vi "Serial_sendot_v7 2.vi"(8 "Numeric 2":i32=20, 9 "VISA resource name":refnum<visa-resource-name>, 10 "Arduino":bool) -> (1 "Array":dbl[](array[numeric]), 2 "Amplitude vs TimeStamp":cluster{dbl[], dbl[]}(graph))   [LabVIEW 2021]
uses:
  Trigger/Control 3.ctl
  Trigger/Control 2.ctl
  <vilib>/Instr/_visa.llb/VISA Configure Serial Port (Instr).vi
  <vilib>/regexp/Match Regular Expression.xnode
panel:
  out "output array 2":dbl[](array[numeric])
  in  "regular expression":string="[0-9]{5,8}"
  out "Final":dbl[](array[numeric])
  out "Signal2":dbl[](array[numeric])
  out "Signal1":dbl[](array[numeric])
  out "whole match 2":string
  in  "write buffer":T1=" {CR}"
  out "return count":u32
  out "read buffer":string
  in  "byte count":T2=1024
  in  "data bits (8)":u16=8 min=5 max=8 step=1
  in  "baud rate (9600)":u32=19200
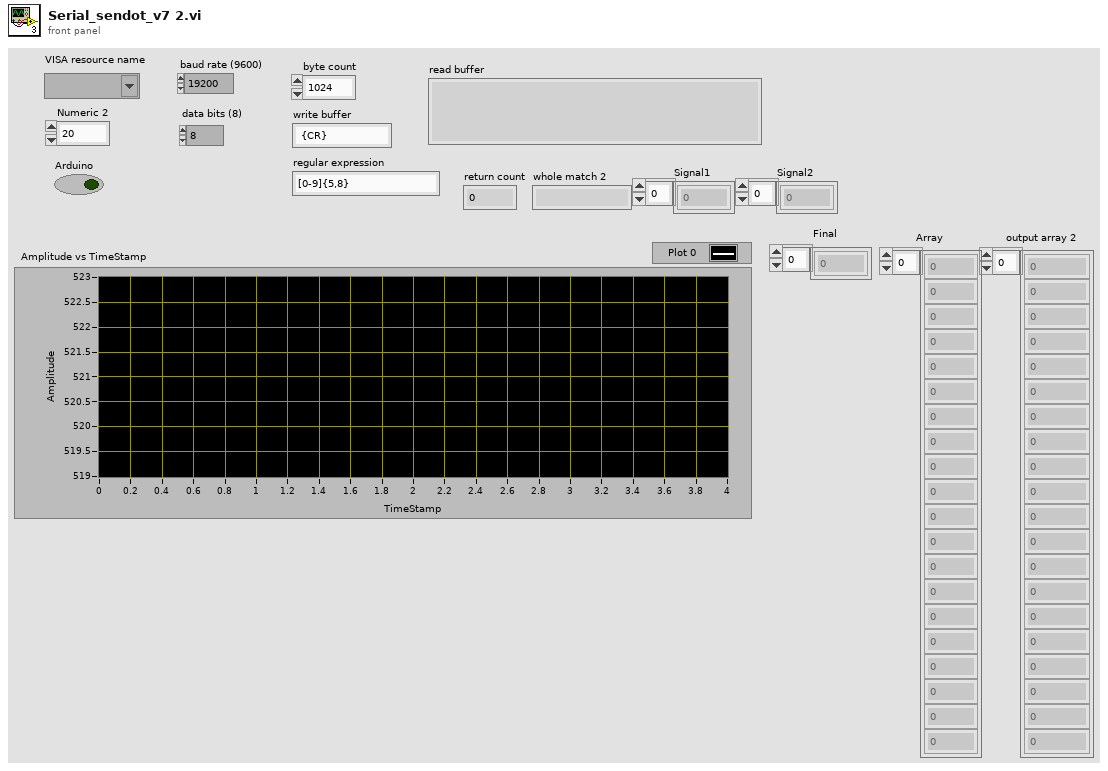
[diagram p1: front panel]
types:
  T1 = typedef "Control 2.ctl" = string
  T2 = typedef "Control 3.ctl" = u32
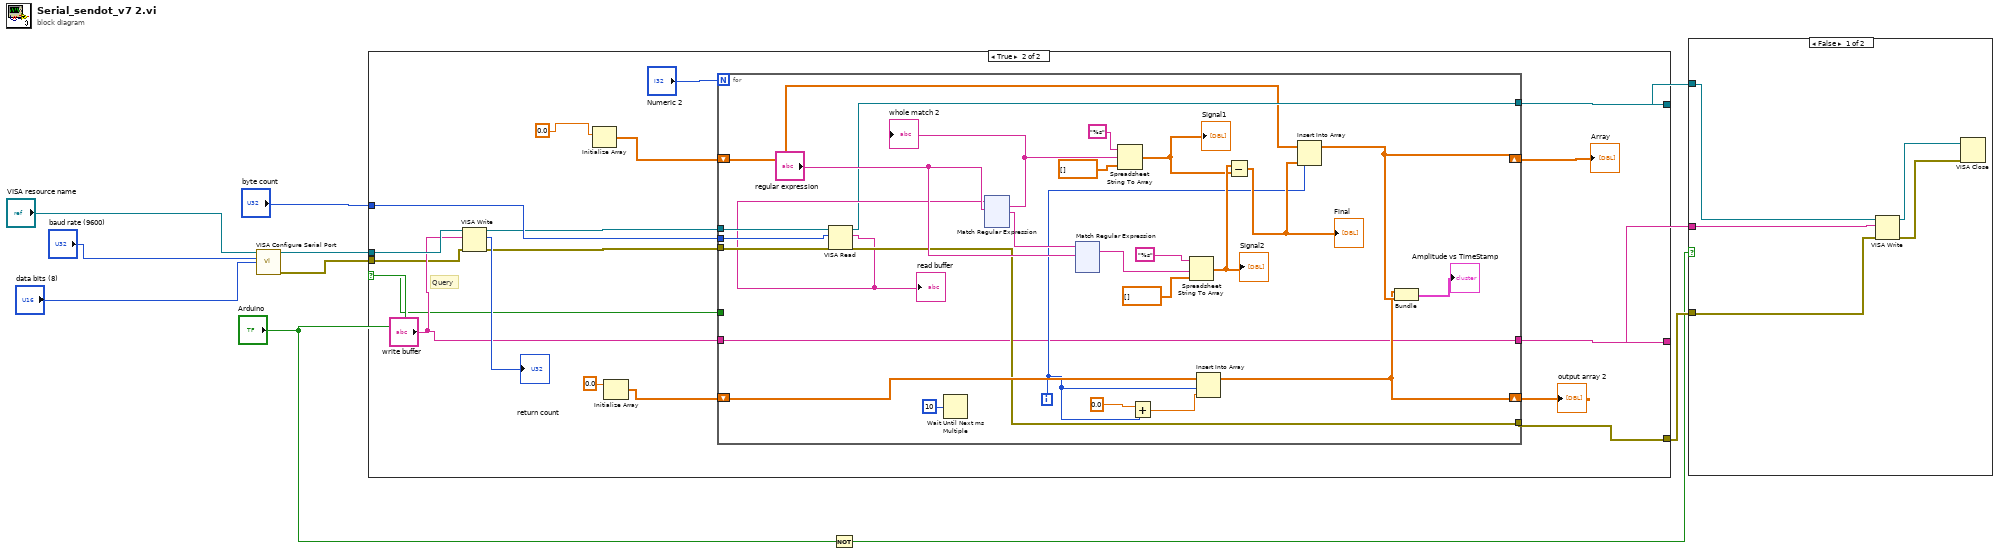
[diagram p0: block diagram]
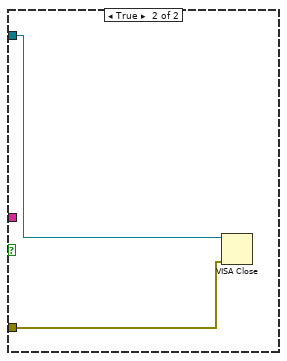
[diagram p2: hidden frame]
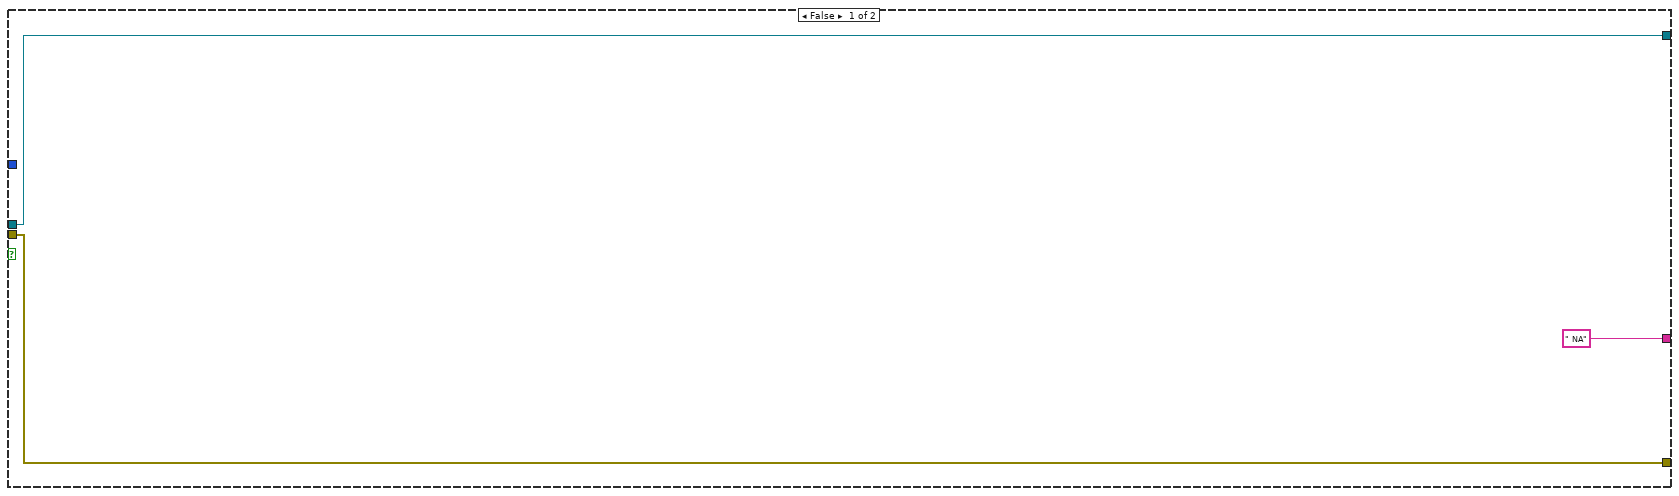
[diagram p3: hidden frame]
diagram:
  n1 = call-poly "VISA Configure Serial Port"("VISA resource name"="VISA resource name", "baud rate (9600)"="baud rate (9600)", "data bits (8)"="data bits (8)") -> ("VISA resource name out"=w2:refnum<visa-resource-name>, "error out"=w1:errorcluster)  [unwired: 11 in]
  n2 = case shown="True" "Arduino" {
    selector: "Arduino" -> [_ w18]
    tunnel: w2 -> [w14 w32]
    tunnel: "byte count" -> [_ w24]
    tunnel: [w12 w22] -> w7
    tunnel: [w14 w19] -> w6
    tunnel: [T1 " NA" ("write buffer") w20] -> w3
    tunnel: w1 -> [w12 w15]
    frame False {
    }
    frame True {
      # "Query"
      n3 = VISA Write(VISA resource name=w32, write buffer="write buffer", error in (no error)=w15) -> (VISA resource name out=w23:refnum<visa-resource-name>, return count=→"return count":u32, error out=w25:errorcluster)
      n4 = Initialize Array(0.0 ("element")) -> (w29:dbl[])  [unwired: 1 in]
      n5 = Initialize Array(0.0 ("element")) -> (w27:dbl[])  [unwired: 1 in]
      n6 = for {
        N: "Numeric 2" -> [_]
        shift-right: [w48] -> w16
        shift-left: w29 -> [w34]
        shift-right: [w42] -> w26
        shift-left: w27 -> [w45]
        tunnel: w25 -> [w41]
        tunnel: w24 -> [w40]
        tunnel: w23 -> [w39]
        tunnel: [w38] -> w22
        tunnel: "write buffer" -> [w36]
        tunnel: [w36] -> w20
        tunnel: [w35] -> w19
        tunnel: w18 -> [_]
        i -> [w43]
        n7 = VISA Read(VISA resource name=w39, byte count=w40, error in (no error)=w41) -> (VISA resource name out=w35:refnum<visa-resource-name>, read buffer=w37:string, error out=w38:errorcluster)  [unwired: 1 out]
        "read buffer" <- w37
        n8 = Wait Until Next ms Multiple(millisecond multiple=u32 10) -> ()  [unwired: 1 out]
        n9 = xnode "Match Regular Expression"("input string"=w37, "regular expression"="regular expression") -> ("whole match"=w56:string, "after match"=w59:string)  [unwired: 4 in, 3 out]
        "whole match 2" <- w56
        n10 = xnode "Match Regular Expression"("input string"=w59, "regular expression"="regular expression") -> ("whole match"=w53:string)  [unwired: 4 in, 4 out]
        n11 = Spreadsheet String To Array(format string="%s", spreadsheet string=w56, array type (2D Dbl)=dbl[] []) -> (array=w51:dbl[])  [unwired: 1 in]
        "Signal1" <- w51
        n12 = Add(x=0.0, y=w43) -> (x+y=w47:dbl)
        n13 = Spreadsheet String To Array(format string="%s", spreadsheet string=w53, array type (2D Dbl)=dbl[] []) -> (array=w52:dbl[])  [unwired: 1 in]
        "Signal2" <- w52
        n14 = Insert Into Array(array=w45, index=w43, new element=w47) -> (w42:dbl[])
        n15 = Subtract(x=w52, y=w51) -> (x-y=w50:dbl[])
        "Final" <- w50
        n16 = Insert Into Array(array=w34, index=w43, new element=w50) -> (w48:dbl[])
        n17 = Bundle(w42, w48) -> (→"Amplitude vs TimeStamp":cluster{dbl[], dbl[]})  [unwired: 1 in]
      }
      "output array 2" <- w26
      "Array" <- w16
    }
  }
  n18 = Not(x="Arduino") -> (.not. x?=w4:bool)
  n19 = case shown="False" w4 {
    tunnel: w7 -> [w294 w299]
    tunnel: w6 -> [w295 w300]
    tunnel: w3 -> [w296 _]
    frame False {
      n20 = VISA Write(VISA resource name=w295, write buffer=w296, error in (no error)=w294) -> (VISA resource name out=w298:refnum<visa-resource-name>, error out=w297:errorcluster)  [unwired: 1 out]
      n21 = VISA Close(VISA resource name=w298, error in (no error)=w297) -> ()  [unwired: 1 out]
    }
    frame True {
      n22 = VISA Close(VISA resource name=w300, error in (no error)=w299) -> ()  [unwired: 1 out]
    }
  }
